vi "Test Get Latest Broadcast Content Correct with Data.vi"(8 "error in (no error)":errorcluster, 11 "Test Case In":refnum<class "Debugger Test.lvclass">) -> (0 "error out":errorcluster, 3 "Test Case Out":refnum<class "Debugger Test.lvclass">)   [LabVIEW 2020]
uses:
  Debugger Test.lvclass
  C:/Program Files (x86)/National Instruments/LabVIEW 2020/vi.lib/Astemes/LUnit/Test Case.lvclass
  source/Debugger/Debugger.lvclass
  C:/Users/anton/Documents/GitHub/triarc-debugger/source/Process/Debug Process.lvclass
  source/Debug Data/Raw Debug Data.ctl
  source/Debug Data/Debug Data.lvclass/Debug Data.ctl
  source/Process/Debug Process.lvclass/Debug Process.ctl
  <vilib>/Astemes/LUnit/Test Case.lvclass/Test Case.ctl
  <vilib>/Astemes/LUnit/LUnit Assertion Result.lvclass/LUnit Assertion Result.ctl
  <vilib>/Astemes/LUnit/LUnit Test Case Result.lvclass/LUnit Test Case Result.ctl
  <vilib>/Astemes/LUnit/LUnit Method Result.lvclass/LUnit Method Result.ctl
  770d5042-3263-43ff-84ad-3943cd9ed827.vi
  <vilib>/AdvancedString/Delimited String to 1D String Array.vi
  source/Process/Public/Lifecycle/Get Lifecycle State.vi
  <vilib>/Astemes/Triarc Framework/Broadcast Event Helpers/Execution timer.vi
  source/Process/Private/SubVIs/Wait for finish.vi
  source/Process/Protected/Messaging/Enqueue Message.vi
  source/Process/Private/SubVIs/Set Lifecycle State.vi
  <vilib>/Astemes/LUnit/Palette/Pass.vi
  <vilib>/Astemes/LUnit/Palette/Fail.vi
  <vilib>/Astemes/LUnit/Compare Variants.vi
  <vilib>/Astemes/LUnit/Describe Comparison.vi
  <vilib>/Astemes/LUnit/Set Assertion Type.vi
  <vilib>/Utility/error.llb/Clear Errors.vi
  <vilib>/Astemes/LUnit/Add test result.vi
  <vilib>/Astemes/LUnit/LUnit Write Passed.vi
  <vilib>/Astemes/LUnit/LUnit Write Message.vi
  <vilib>/Astemes/LUnit/LUnit Write Description.vi
  <vilib>/Astemes/LUnit/Variant to string.vi
  <vilib>/Astemes/LUnit/LUnit Write Assertion Type.vi
  <vilib>/Astemes/LUnit/LUnit Record Assertion Result.vi
  <vilib>/Astemes/LUnit/LUnit Aggregate Assertion Results.vi
  <vilib>/Astemes/LUnit/Assertion Result/LUnit Read Status.vi
  <vilib>/Astemes/LUnit/LUnit Read Message.vi
  <vilib>/Astemes/LUnit/LUnit Read Description.vi
  <vilib>/Astemes/LUnit/Method Result/LUnit Merge Status.vi
  <vilib>/Astemes/LUnit/LUnit Concatenate result strings.vi
  <vilib>/Utility/error.llb/Error Cluster From Error Code.vi
  <vilib>/Astemes/Triarc Framework/Broadcast Event Helpers/Dequeue Broadcast Message.vi
  <vilib>/Utility/Data Type/Get Type Information.vi
  <vilib>/Utility/LVClass/Get LV Class Name.vi
  source/Debug Data/Debug Data.lvclass
  <vilib>/Astemes/LUnit/LUnit Assertion Result.lvclass
  source/Process/Debug Process.lvclass
  <vilib>/Astemes/Triarc Framework/Broadcast Event Helpers/Broadcast Event Helpers.lvlib
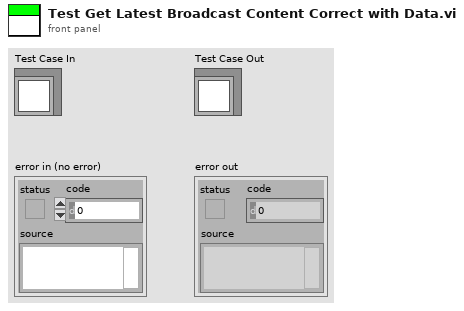
[diagram p1: front panel]
types:
  T1 = typedef "Debug Data.lvclass/Raw Debug Data.ctl" = cluster{"Action":string, "Call Chain":string, "Process":string, "Message":string, "Message Data":variant, "Time":dbl}
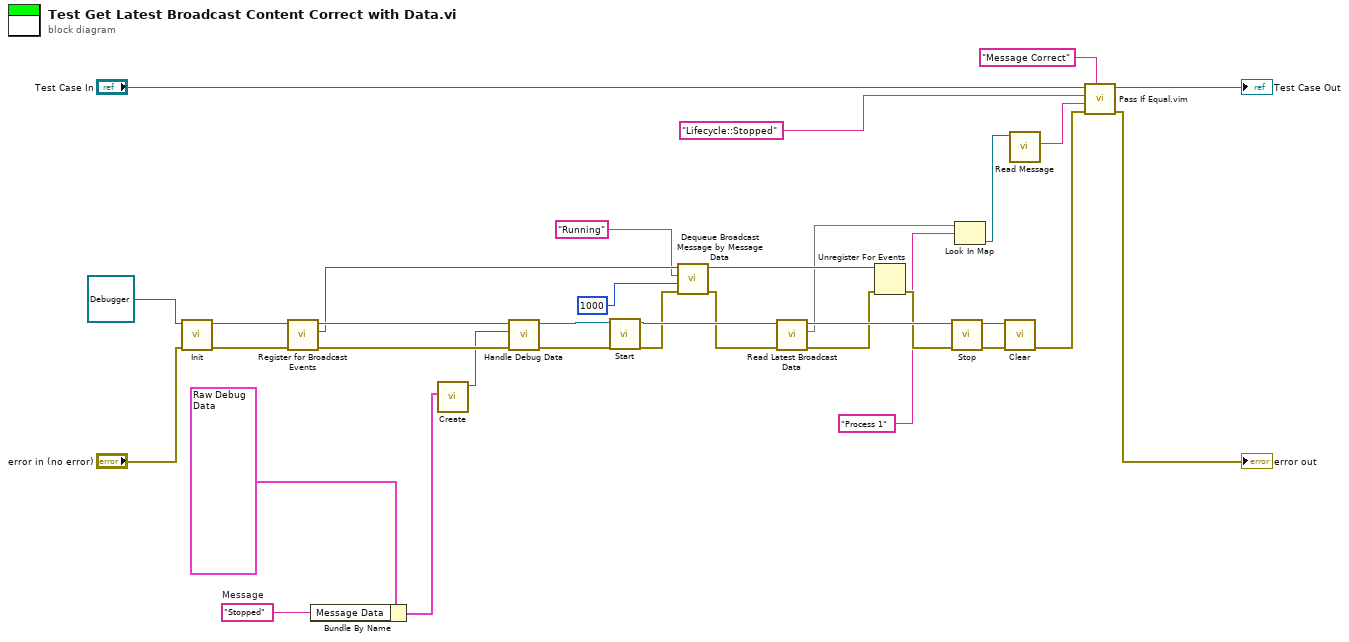
[diagram p0: block diagram]
diagram:
  w3 = "Stopped"  # Message
  n1 = call-dynamic "Init.vi"("error in (no error)"="error in (no error)", "Process In"=refnum<class "Debugger.lvclass"> refnum ("Debug Data Event In 2")) -> ("error out"=w14:errorcluster, "Process Out"=w15:refnum<class "Debugger.lvclass">)  [unwired: 8 in]
  n2 = call "Register for Broadcast Events.vi"("error in (no error)"=w14, "Process In"=w15) -> ("error out"=w31:errorcluster, "Event Registration Refnum Out"=w13:refnum<event-registration>, "Process Out"=w26:refnum<class "Debugger.lvclass">)  [unwired: 7 in]
  n3 = Bundle By Name(cluster=T1 {"Action"="Broadcast", "Call Chain"="", "Process"="Process 1", "Message"="Lifecycle", "Message Data"=variant, "Time"=0.0} ("Debug Data Cluster"), "Message Data"=w3) -> (w1:T1)
  n4 = call "Create.vi"("Debug Data Cluster"=w1) -> ("Debug Data out"=w2:refnum<class "Debug Data.lvclass">)  [unwired: 9 in, 1 out]
  n5 = call-dynamic "Handle Debug Data.vi"("error in (no error)"=w31, "Debug Data.lvclass"=w2, "Debug Data Event In"=w26) -> ("error out"=w30:errorcluster, "Debug Data Event Out"=w17:refnum<class "Debugger.lvclass">)  [unwired: 7 in]
  n6 = call "Start.vi"("error in (no error)"=w30, "Process In"=w17) -> ("error out"=w11:errorcluster, "Process Out"=w16:refnum<class "Debugger.lvclass">)  [unwired: 7 in, 1 out]
  n7 = call <vilib>:"Dequeue Broadcast Message by Message Data.vi"("error in (no error)"=w11, "Timeout (-1)"=1000, "Message Data"="Running", "Event Registration Refnum"=w13) -> ("error out"=w10:errorcluster, "Event Registration Refnum Out"=w12:refnum<event-registration>)  [unwired: 3 in, 3 out]
  n8 = call "Read Latest Broadcast Data.vi"("error in (no error)"=w10, "Debugger In"=w16) -> ("error out"=w21:errorcluster, "Latest Messages"=w7:map{string, refnum<class "Debug Data.lvclass">}, "Debugger Out"=w29:refnum<class "Debugger.lvclass">)  [unwired: 7 in]
  n9 = Unregister For Events(event registration refnum=w12, error in=w21) -> (error out=w20:errorcluster)
  n10 = call "Stop.vi"("error in (no error)"=w20, "Process In"=w29) -> ("error out"=w27:errorcluster, "Process Out"=w28:refnum<class "Debugger.lvclass">)  [unwired: 7 in, 1 out]
  n11 = Look In Map(map=w7, key="Process 1") -> (value=w19:refnum<class "Debug Data.lvclass">)  [unwired: 1 in, 1 out]
  n12 = call-dynamic "Clear.vi"("error in (no error)"=w27, "Process In"=w28) -> ("error out"=w23:errorcluster)  [unwired: 9 in]
  n13 = call "Read Message.vi"("Debug Data in"=w19) -> ("Message"=w6:string)  [unwired: 8 in, 2 out]
  n14 = call "Pass If Equal.vim"("Description"="Message Correct", "error in (no error)"=w23, "Actual"=w6, "Expected"="Lifecycle::Stopped", "LUnit Test Case In"="Test Case In") -> ("error out"=→"error out":errorcluster, "LUnit Test Case Out"=→"Test Case Out":refnum<class "Debugger Test.lvclass">)  [unwired: 5 in]
